vi "FormatFileName.vi"(9 "Subject Id":string, 10 "Base file Name":string, 11 "Folder to save to":path) -> (3 "appended path":path)   [LabVIEW 2016]
doc: "formats filename in the form folder_name/base_subjectId_date_time.csv. if no parameters given, defaults to applciation folder/agression_999_date_time.csv"
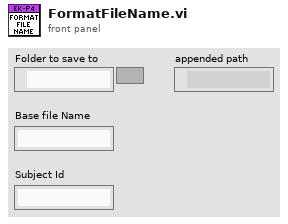
[diagram p1: front panel]
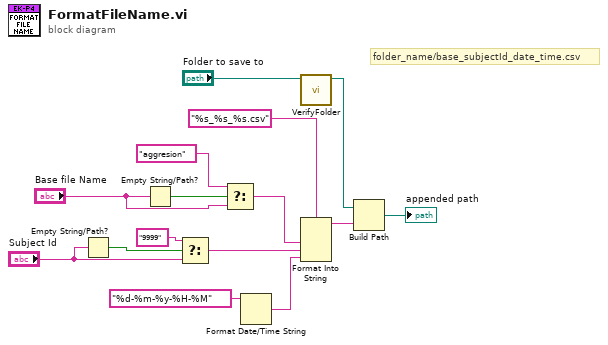
[diagram p0: block diagram]
diagram:
  # "folder_name/base_subjectId_date_time.csv"
  n1 = Empty String/Path?(string/path="Subject Id") -> (empty?=w6:bool)
  n2 = Empty String/Path?(string/path="Base file Name") -> (empty?=w9:bool)
  n3 = Select(t="9999", s=w6, f="Subject Id") -> (s? t:f=w3:string)
  n4 = Select(t="aggresion", s=w9, f="Base file Name") -> (s? t:f=w2:string)
  n5 = Format Date/Time String(time format string (%c)="%d-%m-%y-%H-%M") -> (date/time string=w12:string)  [unwired: 2 in]
  n6 = call "VerifyFolder.vi"("File to save"="Folder to save to") -> ("selected path"=w13:path)  [unwired: 10 in]
  n7 = Format Into String(format string="%s_%s_%s.csv", w2, w3, w12) -> (resulting string=w14:string)  [unwired: 2 in, 1 out]
  n8 = Build Path(base path=w13, name or relative path=w14) -> (appended path=→"appended path":path)
